vi "Add Components to SBOM.vi"(8 "error in (no error)":errorcluster, 10 "Component(s) to add":refnum<class "CycloneDX Component.lvclass">[](array[class]), 11 "CycloneDX SBOM in":refnum<class "CycloneDX JSON.lvclass">) -> (0 "error out":errorcluster, 3 "CycloneDX SBOM out":refnum<class "CycloneDX JSON.lvclass">)   [LabVIEW 2017, in "LabVIEW CycloneDX SBOM.lvlib" / "CycloneDX JSON.lvclass"]
doc: "Adds SBOM components to the SBOM representation (under $.components). As components can be added at multiple levels, this is provided as common functionality, but care should be taken to adhere to the CycloneDX format specification."
uses:
  CycloneDX JSON.lvclass
  CycloneDX Component/CycloneDX Component.lvclass
  C:/LabVIEW Working Directory/labview-cyclonedx-sbom/Source/CycloneDX/CycloneDX JSON/CycloneDX JSON.lvclass
  CycloneDX JSON.lvclass/CycloneDX JSON.ctl
  Read JSON.vi
  Write JSON.vi
  <vilib>/JDP Science/JSONtext/String Subset.vi
  <vilib>/JDP Science/JSONtext/Parsing/Parse Full Path or Item Name.vi
  <vilib>/JDP Science/JSONtext/Next JSON Value.vi
  <vilib>/JDP Science/JSONtext/support/Error Cluster From Code.vi
  <vilib>/JDP Science/JSONtext/Offset/Find Item Locations by Path.vi
  <vilib>/JDP Science/JSONtext/support/Format JSON Array Text.vi
  <vilib>/JDP Science/JSONtext/JSONtext.lvlib
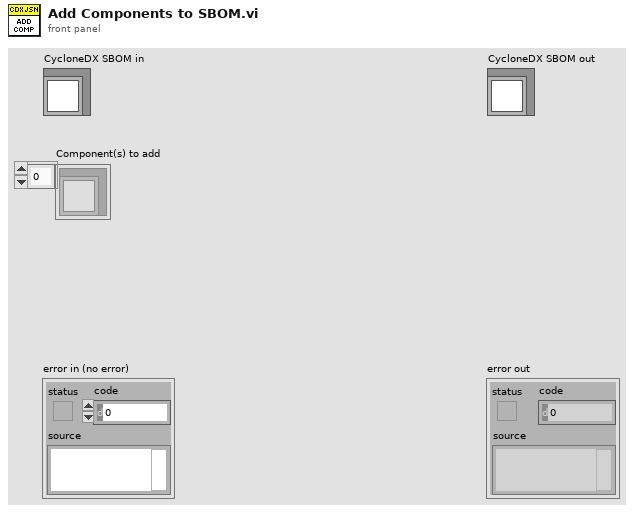
[diagram p1: front panel]
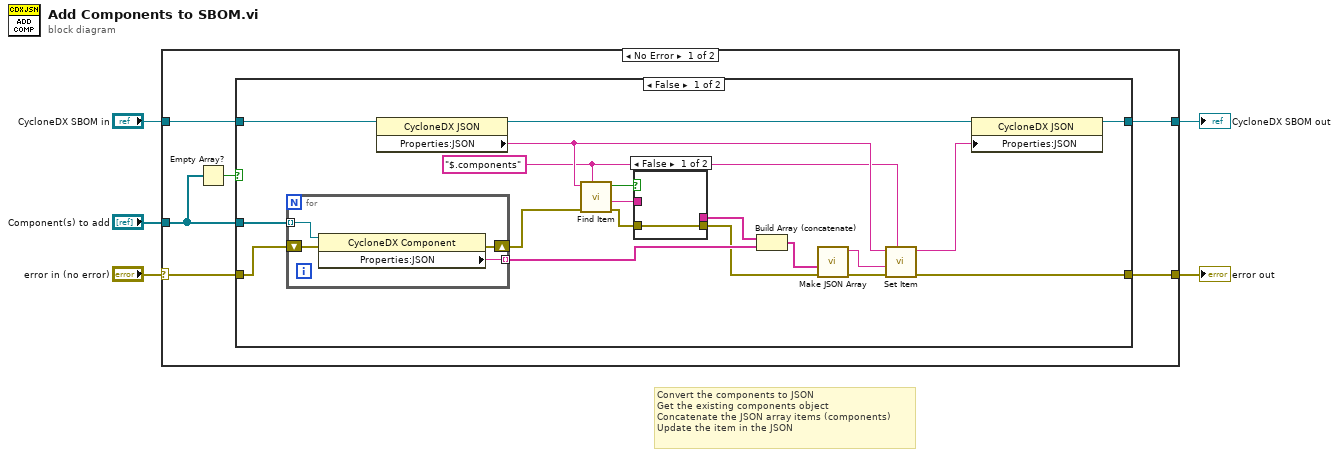
[diagram p0: block diagram]
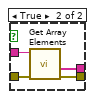
[diagram p2: hidden frame]
diagram:
  # "Convert the components to JSON\nGet the existing components object\nConcatenate the JSON array items (components)\nUpdate the item in the JSON"
  n1 = case shown="No Error" "error in (no error)" {
    selector: "error in (no error)" -> [w9 w43]
    tunnel: [w8 w43] -> w4
    tunnel: [w10 w42] -> w2
    tunnel: "CycloneDX SBOM in" -> [w11 w42]
    tunnel: "Component(s) to add" -> [w6 _]
    frame No Error {
      n2 = Empty Array?(array=w6) -> (empty?=w7:bool)
      n3 = case shown="False" w7 {
        tunnel: w11 -> [w30 w41]
        tunnel: w6 -> [w29 _]
        tunnel: [w27 w41] -> w10
        tunnel: w9 -> [w21 w40]
        tunnel: [w17 w40] -> w8
        frame False {
          w13 = "$.components" ("$Path or Item Name")
          n4 = for {
            tunnel: w29 -> [w39] mode=indexing
            tunnel: [w37] -> w24 mode=indexing
            shift-right: [w36] -> w20
            shift-left: w21 -> [w38]
            n5 = property class="CycloneDX Component"(reference=w39, error in=w38) -> (error out=w36:errorcluster, "Properties:JSON"=w37:string)  [unwired: 1 out]
          }
          n6 = property class="CycloneDX JSON"(reference=w30) -> (reference out=w28:refnum<class "CycloneDX JSON.lvclass">, "Properties:JSON"=w15:string)  [unwired: 1 in, 1 out]
          n7 = call <vilib>:"Find Item.vi"("$Path or Item Name"=w13, "error in (no error)"=w20, "JSON"=w15) -> ("error out"=w22:errorcluster, "<JSON>"=w26:string, "Found"=w12:bool)  [unwired: 5 in, 1 out]
          n8 = case shown="False" w12 {
            tunnel: w26 -> [_ w35]
            tunnel: [_ w34] -> w25
            tunnel: w22 -> [w31 w33]
            tunnel: [w31 w32] -> w19
            frame False {
            }
            frame True {
              n9 = call <vilib>:"Get Array Elements.vi"("error in (no error)"=w33, "JSON"=w35) -> ("error out"=w32:errorcluster, "<JSON>"=w34:string[])  [unwired: 7 in, 1 out]
            }
          }
          n10 = Build Array (concatenate)(w25, w24) -> (w23:string[])
          n11 = call <vilib>:"Make JSON Array.vi"("error in (no error)"=w19, "JSON Elements"=w23) -> ("error out"=w18:errorcluster, "<JSON>"=w14:string)  [unwired: 8 in]
          n12 = call <vilib>:"Set Item.vi"("$Path or Item Name"=w13, "error in (no error)"=w18, "JSON to Insert"=w14, "JSON"=w15) -> ("error out"=w17:errorcluster, "<JSON>"=w16:string)  [unwired: 4 in, 1 out]
          n13 = property class="CycloneDX JSON"(reference=w28, "Properties:JSON"=w16) -> (reference out=w27:refnum<class "CycloneDX JSON.lvclass">)  [unwired: 1 in, 1 out]
        }
        frame True {
        }
      }
    }
    frame Error {
    }
  }
  "error out" <- w4
  "CycloneDX SBOM out" <- w2
